vi "Initialize SPI.vi"(5 "TestSocketName":string, 11 "error in":errorcluster) -> (4 "Tasks":T1, 6 "rate":dbl, 15 "error out":errorcluster)   [LabVIEW 2023, in "SPI.lvlib"]
uses:
  SPI.lvlib
  Tasks.ctl
  <vilib>/DAQmx/create/channels.llb/DAQmx Create Channel (DO-Digital Output).vi
  <vilib>/DAQmx/configure/timing.llb/DAQmx Timing (Sample Clock).vi
  <vilib>/DAQmx/create/channels.llb/DAQmx Create Channel (DI-Digital Input).vi
  <vilib>/DAQmx/create/channels.llb/DAQmx Create Channel (CO-Pulse Generation-Frequency).vi
  <vilib>/DAQmx/configure/timing.llb/DAQmx Timing (Implicit).vi
  <resource>/objmgr/daqmx.rc
panel:
  out "MISO task":refnum<k21>
  out "MOSI task":refnum<k21>
  out "CLK task":refnum<k21>
  out "CS task":refnum<k21>
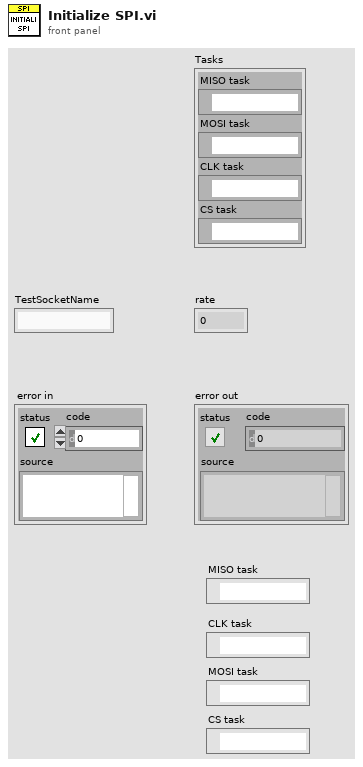
[diagram p1: front panel]
types:
  T1 = typedef "SPI.lvlib/Tasks.ctl" = cluster{"MISO task":refnum<k21>, "MOSI task":refnum<k21>, "CLK task":refnum<k21>, "CS task":refnum<k21>}
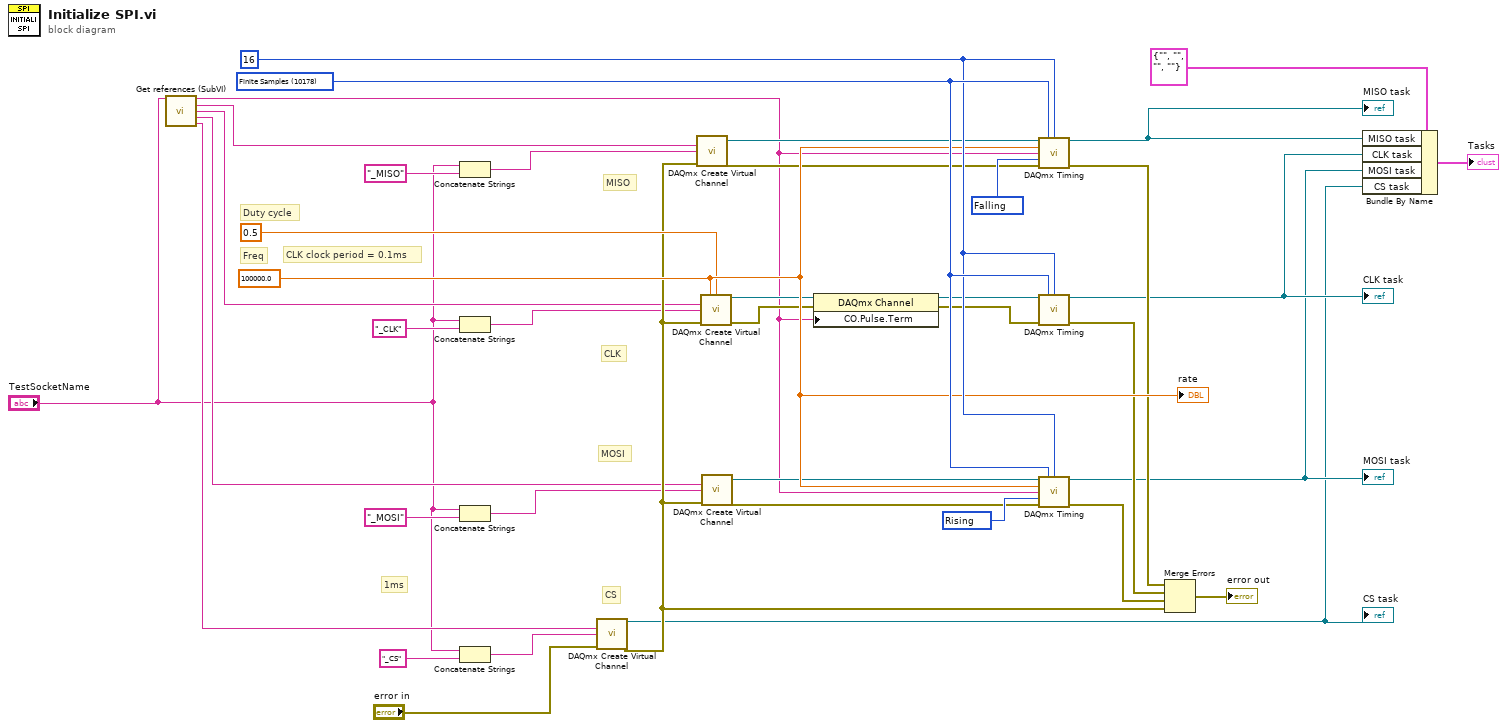
[diagram p0: block diagram]
diagram:
  w38 = 100000.0 ("rate")
  w32 = 10280 items=["Rising"=10280, "Falling"=10171] ("active edge")
  w31 = 10171 items=["Rising"=10280, "Falling"=10171] ("active edge")
  w39 = 16 ("samples per channel")
  w40 = 10178 items=["Finite Samples"=10178, "Continuous Samples"=10123, "Hardware Timed Single Point"=12522] ("sample mode")
  # "CLK clock period = 0.1ms"
  # "Duty cycle"
  # "Freq"
  # "1ms"
  # "CS"
  # "MOSI"
  # "CLK"
  # "MISO"
  n1 = call "Get references (SubVI).vi"("TestSocketName in"="TestSocketName") -> ("MISO CO.Pulse.Term"=w3:tag, "MISO"=w2:tag, "CLK"=w6:tag, "MOSI"=w5:tag, "CS"=w4:tag)  [unwired: 10 in]
  n2 = Concatenate Strings("TestSocketName", "_MISO" ("name to assign")) -> (w14:string)
  n3 = Concatenate Strings("TestSocketName", "_CLK" ("name to assign")) -> (w16:string)
  n4 = Concatenate Strings("TestSocketName", "_MOSI" ("name to assign")) -> (w18:string)
  n5 = Concatenate Strings("TestSocketName", "_CS" ("name to assign")) -> (w21:string)
  n6 = call-poly <vilib>:"DAQmx Create Virtual Channel.vi"("lines"=w4, "name to assign"=w21, "error in"="error in") -> ("task out"=w9:refnum<k21>, "error out"=w26:errorcluster)  [unwired: 11 in]
  "CS task" <- w9
  n7 = call-poly <vilib>:"DAQmx Create Virtual Channel.vi"("lines"=w2, "name to assign"=w14, "error in"=w26) -> ("task out"=w27:refnum<k21>, "error out"=w28:errorcluster)  [unwired: 11 in]
  n8 = call-poly <vilib>:"DAQmx Create Virtual Channel.vi"("frequency"=w38, "duty cycle"=0.5, "counter"=w6, "name to assign"=w16, "error in"=w26) -> ("task out"=w34:refnum<k21>, "error out"=w35:errorcluster)  [unwired: 9 in]
  n9 = call-poly <vilib>:"DAQmx Create Virtual Channel.vi"("lines"=w5, "name to assign"=w18, "error in"=w26) -> ("task out"=w29:refnum<k21>, "error out"=w30:errorcluster)  [unwired: 11 in]
  n10 = property class="DAQmx Channel"(reference=w34, error in=w35, "CO.Pulse.Term"=w3) -> (reference out=w36:refnum<k21>, error out=w37:errorcluster)
  n11 = call-poly <vilib>:"DAQmx Timing.vi"("task/channels in"=w27, "sample mode"=w40, "samples per channel"=w39, "rate"=w38, "source"=w3, "active edge"=w31, "error in"=w28) -> ("task out"=w12:refnum<k21>, "error out"=w25:errorcluster)  [unwired: 7 in]
  "MISO task" <- w12
  n12 = call-poly <vilib>:"DAQmx Timing.vi"("task/channels in"=w36, "sample mode"=w40, "samples per channel"=w39, "error in"=w37) -> ("task out"=w11:refnum<k21>, "error out"=w24:errorcluster)  [unwired: 10 in]
  "CLK task" <- w11
  n13 = call-poly <vilib>:"DAQmx Timing.vi"("task/channels in"=w29, "sample mode"=w40, "samples per channel"=w39, "rate"=w38, "source"=w3, "active edge"=w32, "error in"=w30) -> ("task out"=w10:refnum<k21>, "error out"=w23:errorcluster)  [unwired: 7 in]
  "MOSI task" <- w10
  n14 = Merge Errors(w25, w24, w23, w26) -> (→"error out":errorcluster)
  n15 = Bundle By Name(cluster=T1 {"MISO task"="", "MOSI task"="", "CLK task"="", "CS task"=""}, "MISO task"=w12, "CLK task"=w11, "MOSI task"=w10, "CS task"=w9) -> (→"Tasks":T1)
  "rate" <- w38
